vi "{{Msg}}.vi"(6 "Error":errorcluster, 7 "Actor Layer":refnum<class "Actor Layer.lvclass">, 9 "Payload":T1, 10 "Msg Attribs":T11 {"Listen Absolute Time" format="%<%x %.3X>T"; "Tell Absolute Time" format="%<%x %.3X>T"}, 11 "Actor":T2) -> (1 "Payload":T1, 2 "Msg Attribs":T11 {"Listen Absolute Time" format="%<%x %.3X>T"; "Tell Absolute Time" format="%<%x %.3X>T"}, 3 "Actor":T2, 4 "Error":errorcluster, 5 "Actor Layer":refnum<class "Actor Layer.lvclass">)   [LabVIEW 2020, in "_Template.lvlib" / "{{Actor}}.lvlib" / "Actor Layer.lvclass"]
uses:
  Actor Layer.lvclass
  Actor Layer.lvclass/Actor Layer.ctl
  jettl/jettl/Origin.ctl
  jettl/jettl/jettl.lvlib
  jettl/jettl/Lifecycle.ctl
  jettl/jettl/Msg Attribs.ctl
  jettl/jettl/Msg/Msg.lvclass
  jettl/jettl/Msg.ctl
  jettl/jettl/Post Setup.ctl
  jettl/jettl/Pre Setup.ctl
  jettl/jettl/Msg Set.ctl
  jettl/jettl/Actor Attribs.ctl
  jettl/jettl/Children.ctl
  jettl/jettl/Actor.ctl
  jettl/jettl/Layer Type.ctl
  jettl/jettl/Layer Attribs.ctl
  jettl/jettl/Layer Map.ctl
  jettl/jettl/Actor Layer/Actor Layer.lvclass
  jettl/jettl/Implemented Map.ctl
  {{Msg}}/Payload.ctl
  {{Msg}}/{{Msg}}.lvlib
panel:
  # "This front panel should not be manipulated."
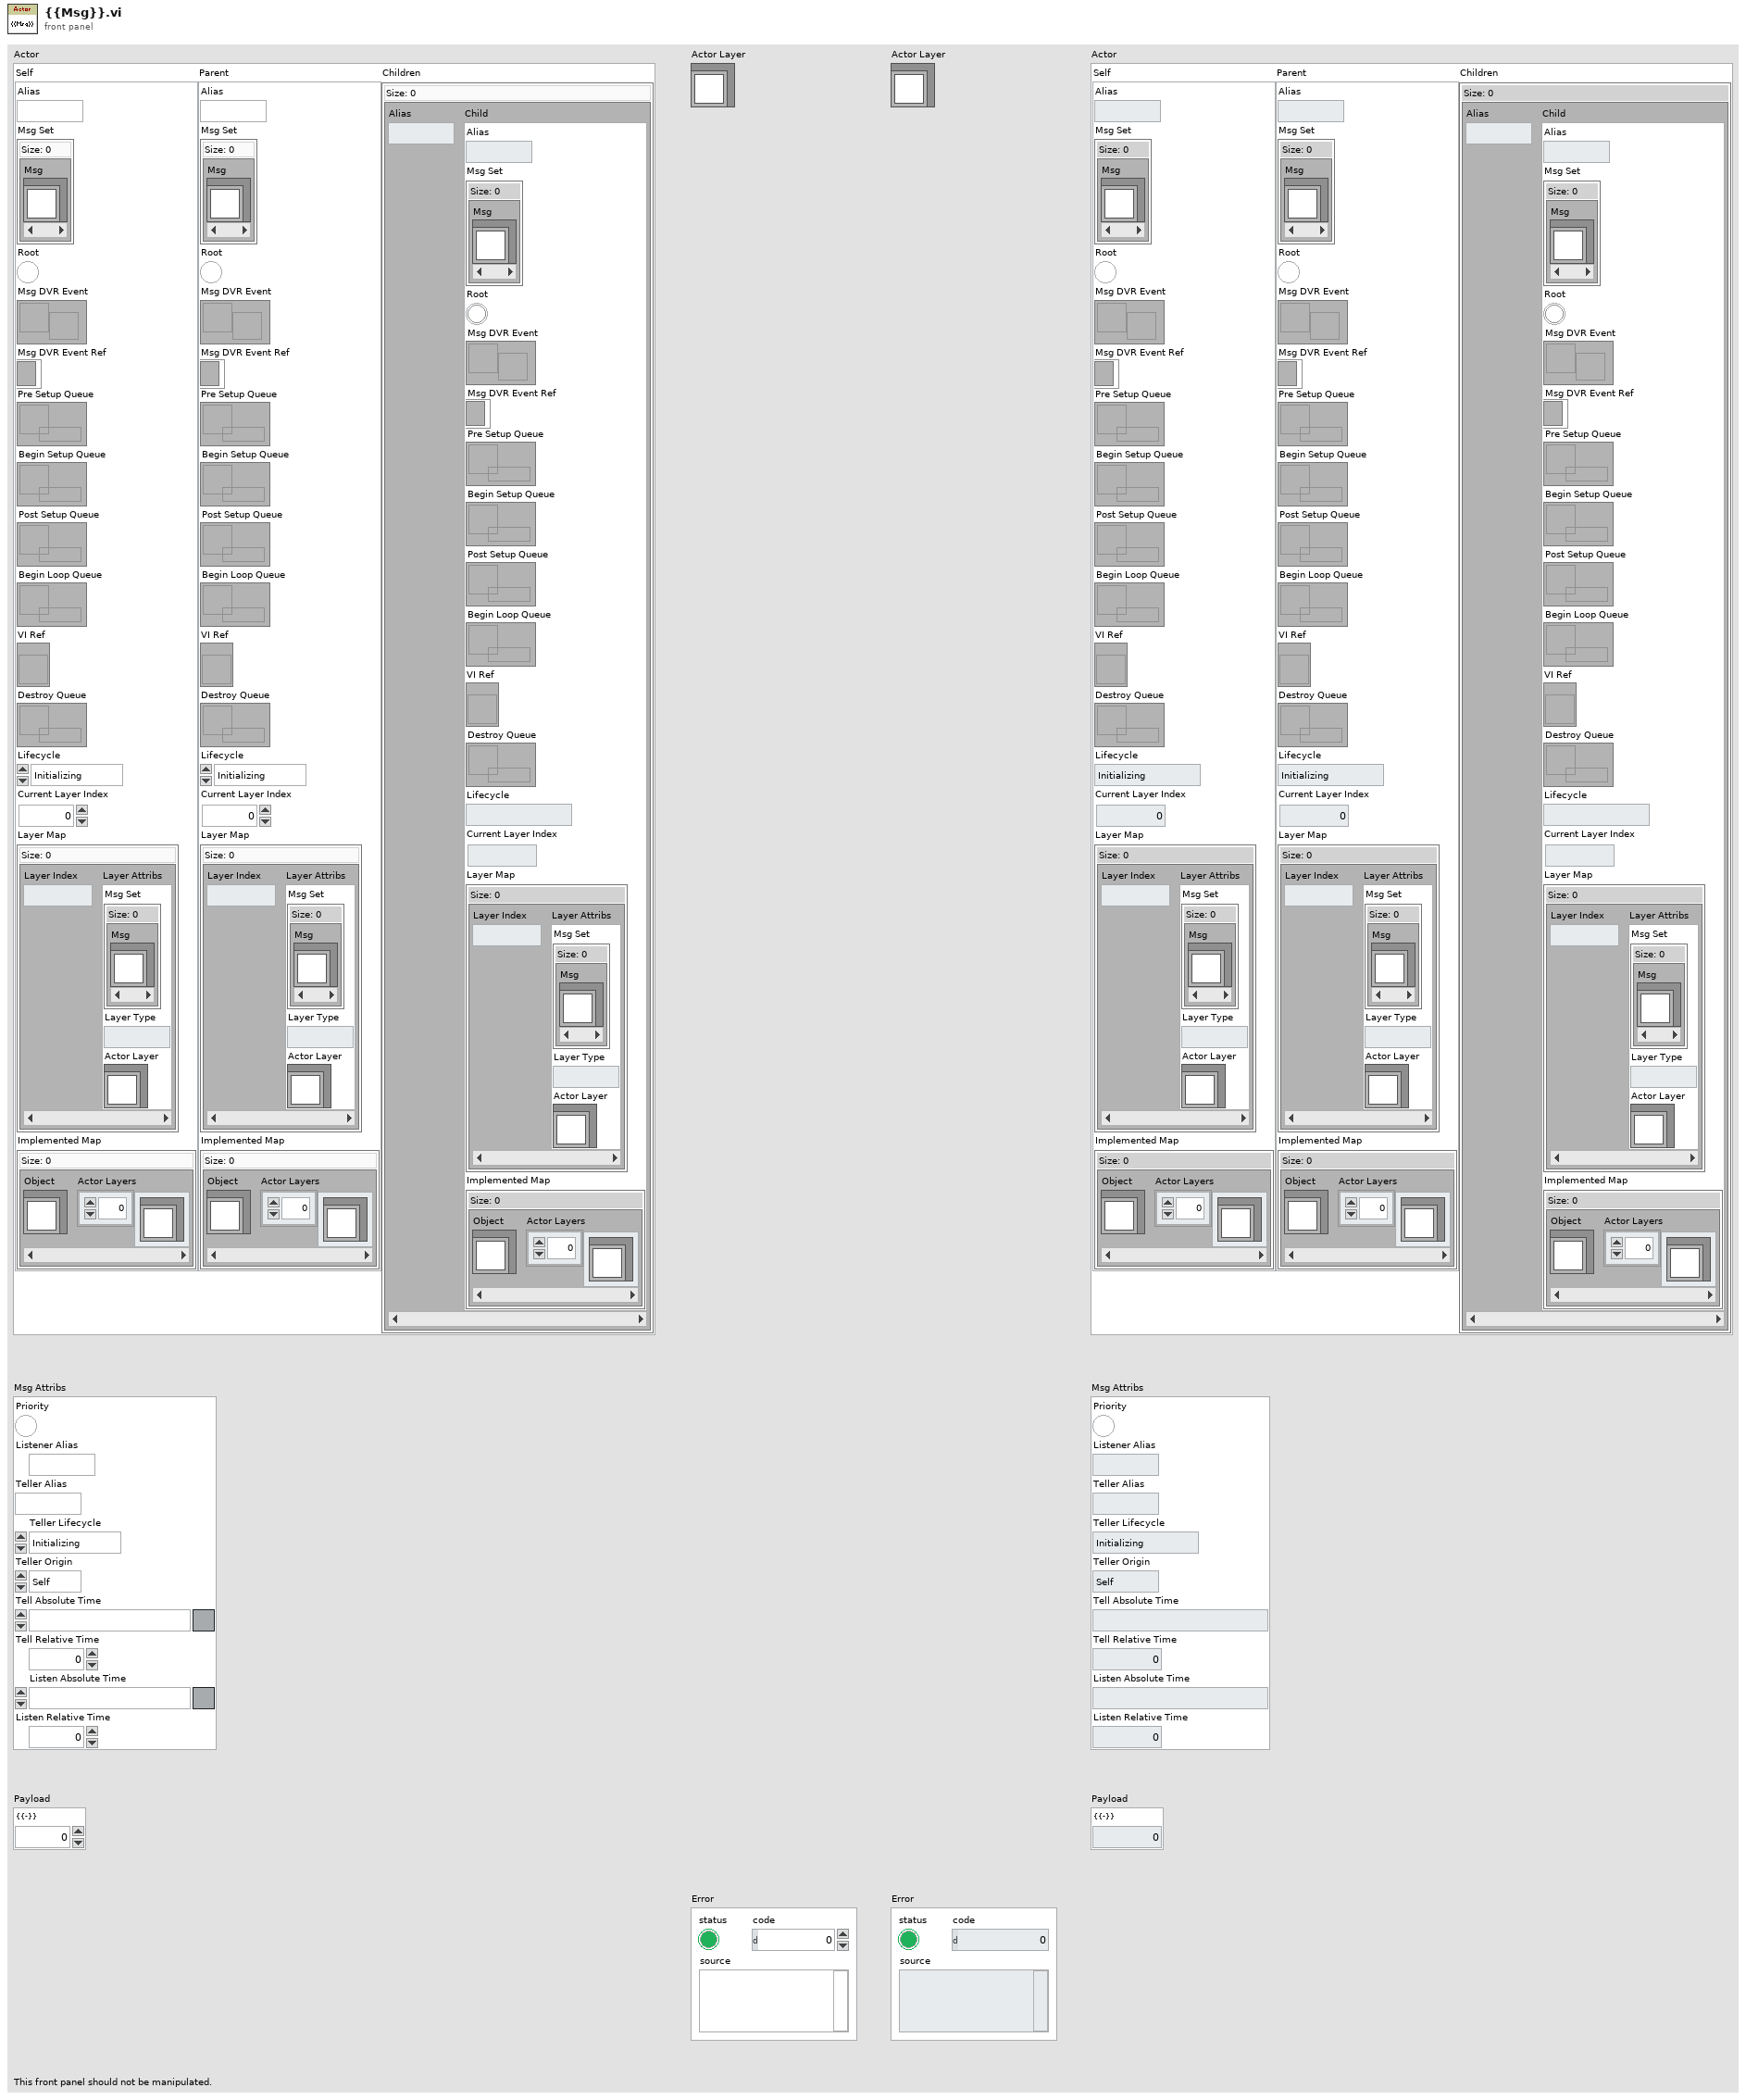
[diagram p1: front panel]
types:
  T1 = typedef "_Template.lvlib/{{Msg}}.lvlib/Payload.ctl" = cluster{"{{-}}":u8}
  T2 = typedef "jettl.lvlib/Actor.ctl" = cluster{"Self":T3, "Parent":T3, "Children":T10}
  T3 = typedef "jettl.lvlib/Actor Attribs.ctl" = cluster{"Alias":string, "Msg Set":T4, "Root":bool, "Msg DVR Event":refnum<user-event>, "Msg DVR Event Ref":refnum<event-registration>, "Pre Setup Queue":refnum<queue>, "Begin Setup Queue":refnum<queue>, "Post Setup Queue":refnum<queue>, "Begin Loop Queue":refnum<queue>, "VI Ref":refnum<vi>, "Destroy Queue":refnum<queue>, "Lifecycle":T5, "Current Layer Index":i32, "Layer Map":T6, "Implemented Map":T9}
  T4 = typedef "jettl.lvlib/Msg Set.ctl" = set{refnum<class "Msg.lvclass">}
  T5 = typedef "jettl.lvlib/Lifecycle.ctl" = enum16{"Initializing", "Setting Up", "Starting", "Running", "Stopping", "Tearing Down", "Terminated"}
  T6 = typedef "jettl.lvlib/Layer Map.ctl" = map{i32, T7}
  T7 = typedef "jettl.lvlib/Layer Attribs.ctl" = cluster{"Msg Set":T4, "Layer Type":T8, "Actor Layer":refnum<class "Actor Layer.lvclass">}
  T8 = typedef "jettl.lvlib/Layer Type.ctl" = enum16{"Base", "InnerGlobal", "InnerLocal", "Outer"}
  T9 = typedef "jettl.lvlib/Implemented Map.ctl" = map{refnum<class>, refnum<class "Actor Layer.lvclass">[]}
  T10 = typedef "jettl.lvlib/Children.ctl" = map{string, T3}
  T11 = typedef "jettl.lvlib/Msg Attribs.ctl" = cluster{"Priority":bool, "Listener Alias":string, "Teller Alias":string, "Teller Lifecycle":T5, "Teller Origin":T12, "Tell Absolute Time":timestamp, "Tell Relative Time":dbl, "Listen Absolute Time":timestamp, "Listen Relative Time":dbl}
  T12 = typedef "jettl.lvlib/Origin.ctl" = enum16{"Self", "Parent", "Child"}
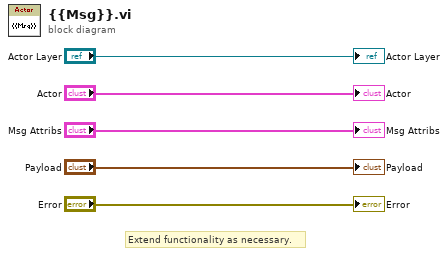
[diagram p0: block diagram]
diagram:
  # "Extend functionality as necessary."
  "Actor Layer" <- "Actor Layer"
  "Error" <- "Error"
  "Msg Attribs" <- "Msg Attribs"
  "Actor" <- "Actor"
  "Payload" <- "Payload"
